vi "IMU Data Loop (RT RHIT's conflicted copy 2012-05-01).vi"() -> ()   [LabVIEW 2011]
uses:
  <vilib>/robotics/Controls/Compass Indicator/Compass Indicator.xctl
  <vilib>/Platform/TimedLoop/XDataNode/timing_clust.ctl
  <vilib>/Platform/TimedLoop/XDataNode/nitl_modes.ctl
  <vilib>/Platform/TimedLoop/XDataNode/wakeup.ctl
  <vilib>/Platform/TimedLoop/XDataNode/XDataNode.xnode
  <instrlib>/MicroStrain 3DM-GX1/MicroStrain 3DM-GX1.lvlib
  <vilib>/Platform/TimedLoop/XDataNode/XDNodeRunTimeDep.lvlib
panel:
  out "Waveform Chart 2":T1(graph)
  out "Waveform Chart":cluster{"Roll":dbl, "Pitch":dbl, "Yaw":dbl}(graph)
  in  "stop?":bool
  out "IMU Data":T2 {"Quaternion" format="%#.4g"; "Angular Rate"."Z-Axis Angular Rate" format="%#.4g"; "Angular Rate"."Y-Axis Angular Rate" format="%#.4g"; "Angular Rate"."X-Axis Angular Rate" format="%#.4g"; "Acceleration"."X-Axis Acceleration" format="%#.4g"; "Acceleration"."Y-Axis Acceleration" format="%#.4g"; "Acceleration"."Z-Axis Acceleration" format="%#.4g"; "Magnetic Field"."X-Axis Magnetic Field" format="%#.4g"; "Magnetic Field"."Y-Axis Magnetic Field" format="%#.4g"; "Magnetic Field"."Z-Axis Magnetic Field" format="%#.4g"; "Orientation Matrix" format="%#.4g"; "Position"."Yaw" format="%#.2f"; "Position"."Pitch" format="%#.1f"; "Position"."Roll" format="%#.1f"}
  in  "North Offset":dbl
  out "Compass Indicator":dbl(xcontrol)
  out "error out":errorcluster
  in  "Baud Rate":u32(ring)=115200 items=["19200"=19200, "38400"=38400, "115200"=115200]
  in  "Test Mode":bool
  in  "VISA resource name":refnum<visa-resource-name>="COM13"
  in  "Configure":bool
  out "Error Display":errorcluster
  in  "Enable Gyro-Stabilization (Enable)":bool=TRUE
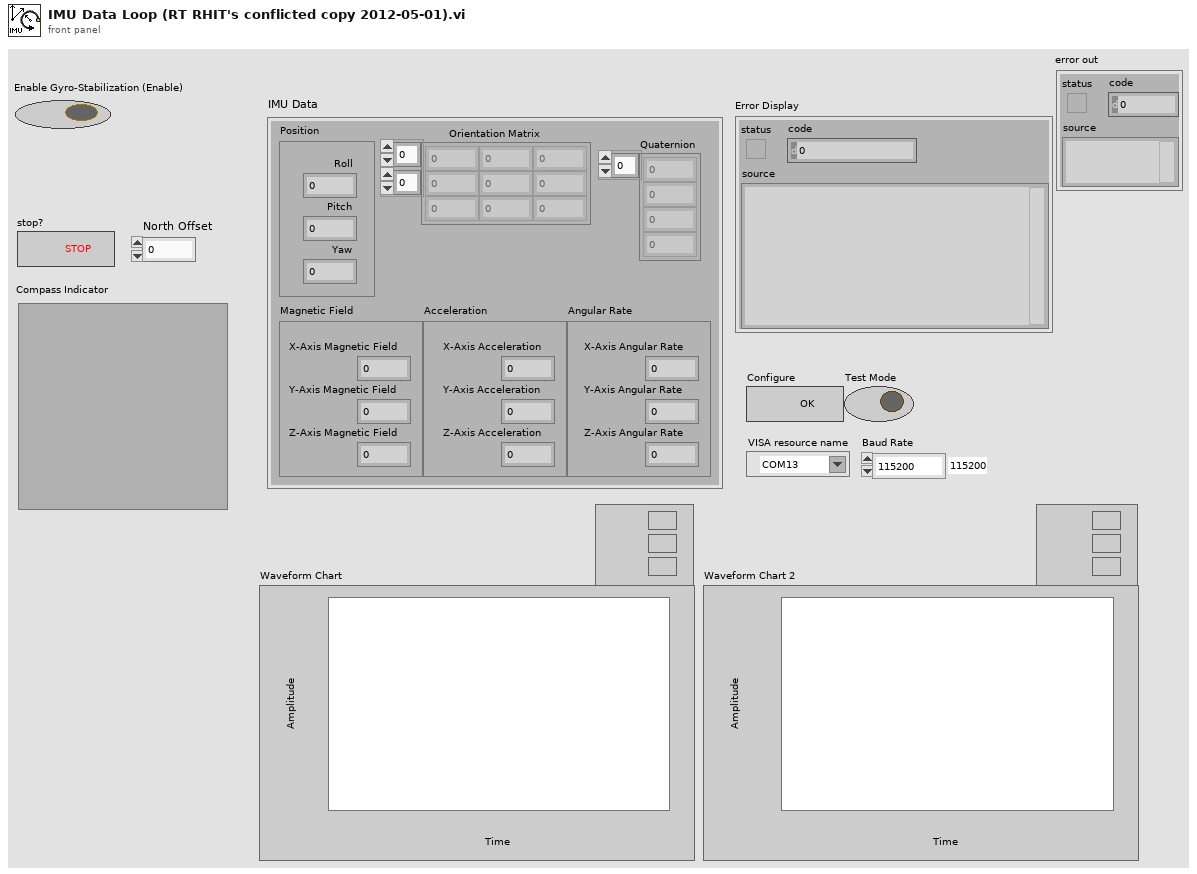
[diagram p1: front panel]
types:
  T1 = cluster{"X-Axis Magnetic Field":dbl, "Y-Axis Magnetic Field":dbl, "Z-Axis Magnetic Field":dbl}
  T2 = cluster{"Position":cluster{"Roll":dbl, "Pitch":dbl, "Yaw":dbl}, "Orientation Matrix":dbl[][], "Magnetic Field":cluster{"Z-Axis Magnetic Field":dbl, "Y-Axis Magnetic Field":dbl, "X-Axis Magnetic Field":dbl}, "Acceleration":cluster{"Z-Axis Acceleration":dbl, "Y-Axis Acceleration":dbl, "X-Axis Acceleration":dbl}, "Angular Rate":cluster{"X-Axis Angular Rate":dbl, "Y-Axis Angular Rate":dbl, "Z-Axis Angular Rate":dbl}, "Quaternion":dbl[]}
  T3 = typedef "XDNodeRunTimeDep.lvlib/timing_clust.ctl" = cluster{"Expected End [f-1]":u64, "Actual End [f-1]":u64, "Finished Late? [f-1]":bool, "Expected End [i-1]":u64, "Actual End [i-1]":u64, "Finished Late? [i-1]":bool, "Expected Start [i]":u64, "Actual Start [i]":u64, "Expected Start [f]":u64, "Actual Start [f]":u64, "Source Name":string, "Structure Name":string, "Period":i64, "Deadline":i64, "Offset":i64, "Start":i64, "Priority":i32, "Timeout":i32, "Mode":T4, "Wakeup Reason":T5, "Error":errorcluster, "Source Type":string, "Secondary Source Type":string, "Global End Time":u64, "Global Start Time":u64, "Frame Duration":u64, "Iteration Duration":u64, "Assigned CPU":i32, "I/O Scan Engine Mode":u32}
  T4 = typedef "XDNodeRunTimeDep.lvlib/nitl_modes.ctl" = enum32{"No Change", "Process missed periods, maintain original phase", "Discard missed periods, maintain original phase", "Process missed periods, ignore original phase", "Discard missed periods, ignore original phase"}
  T5 = typedef "XDNodeRunTimeDep.lvlib/wakeup.ctl" = enum32{"Normal", "Aborted", "Asynchronous wakeup", "Timing source error", "Timed loop error", "Timeout"}
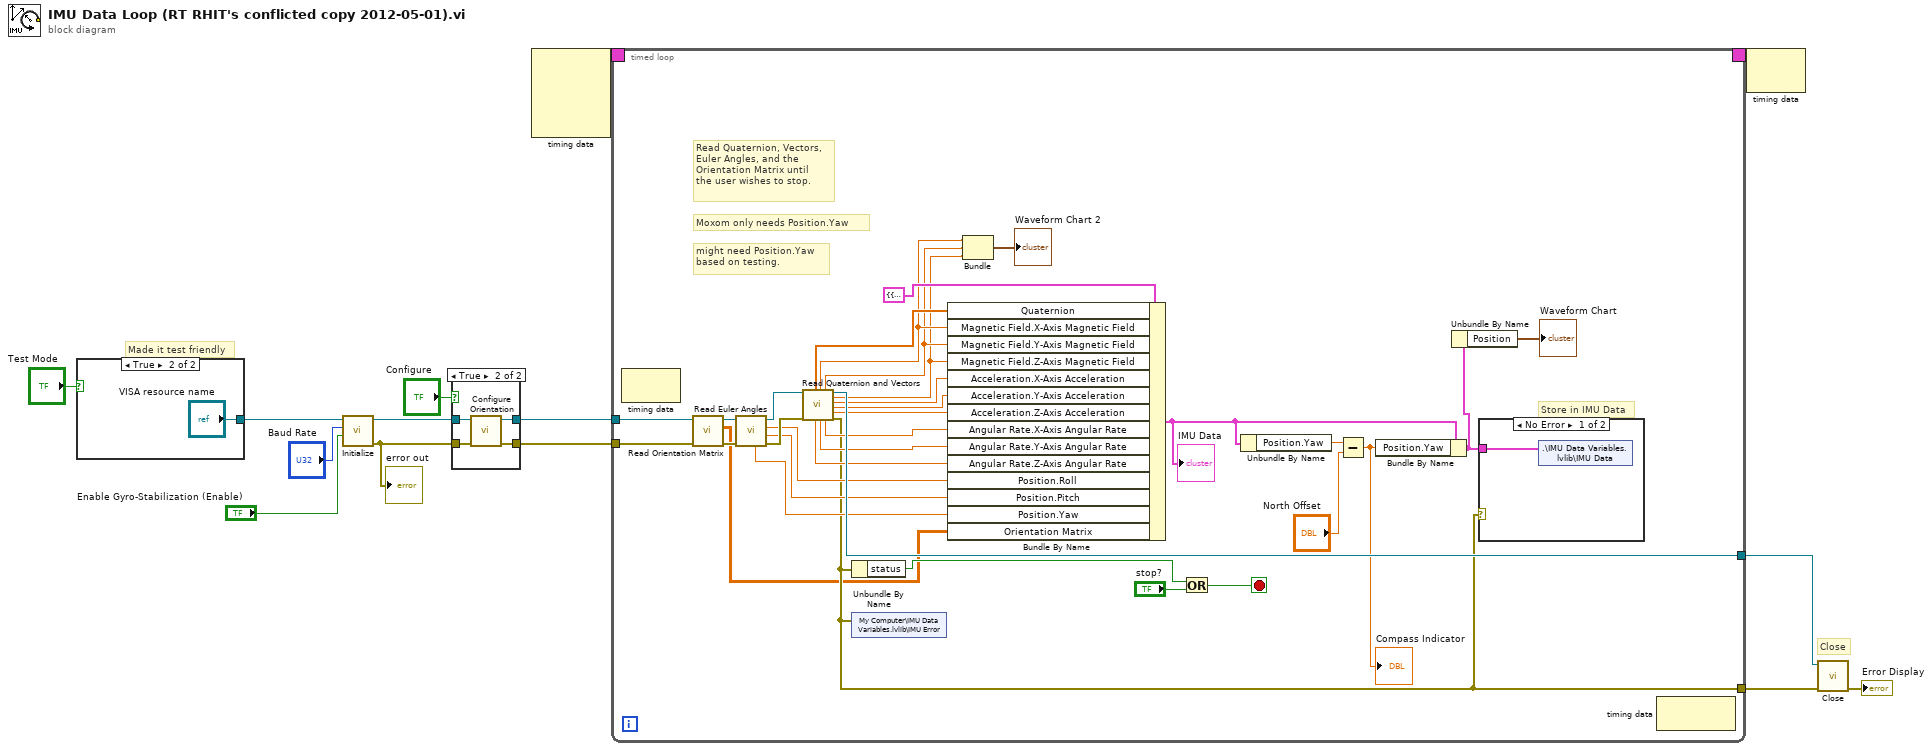
[diagram p0: block diagram]
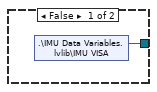
[diagram p3: hidden frame]
diagram:
  # "Made it test friendly"
  # "Close"
  n1 = case shown="True" "Test Mode" {
    tunnel: [w15 "VISA resource name"] -> w7
    frame False {
      n2 = shared-variable ".\\IMU Data Variables.lvlib\\IMU VISA"() -> (w15:refnum<visa-resource-name>)  [unwired: 1 in, 1 out]
    }
    frame True {
    }
  }
  n3 = call <instrlib>:"Initialize.vi"("Enable Gyro-Stabilization (True)"="Enable Gyro-Stabilization (Enable)", "Baud Rate (38400)"="Baud Rate", "VISA resource name"=w7) -> ("error out"=w11:errorcluster, "VISA resource name out"=w12:refnum<visa-resource-name>)  [unwired: 7 in]
  "error out" <- w11
  n4 = case shown="True" "Configure" {
    tunnel: w12 -> [w18 w22]
    tunnel: w11 -> [w17 w21]
    tunnel: [w18 w20] -> w2
    tunnel: [w17 w19] -> w1
    frame False {
    }
    frame True {
      n5 = call <instrlib>:"Configure Orientation.vi"("error in (no error)"=w21, "VISA resource name"=w22) -> ("error out"=w19:errorcluster, "VISA resource name out"=w20:refnum<visa-resource-name>)  [unwired: 8 in]
    }
  }
  n6 = node-c288() -> (w14:T3)  [unwired: 4 in]
  n7 = timed-loop {
    tunnel: [w36] -> w10
    tunnel: [w53] -> w9
    timing: w14 -> [_]
    timing-out: [_] -> w13
    tunnel: w2 -> [w30]
    tunnel: w1 -> [w29]
    stop <- w51 stop-if-true
    # "Moxom only needs Position.Yaw"
    # "Store in IMU Data"
    # "might need Position.Yaw\nbased on testing."
    # "Read Quaternion, Vectors,\nEuler Angles, and the\nOrientation Matrix until\nthe user wishes to stop."
    n8 = node-c288() -> ()  [unwired: 1 in, 1 out]
    n9 = call <instrlib>:"Read Orientation Matrix.vi"("error in (no error)"=w29, "VISA resource name"=w30) -> ("error out"=w54:errorcluster, "Orientation Matrix"=w35:dbl[][], "VISA resource name out"=w55:refnum<visa-resource-name>)  [unwired: 7 in]
    n10 = call <instrlib>:"Read Euler Angles.vi"("error in (no error)"=w54, "VISA resource name"=w55) -> ("error out"=w49:errorcluster, "Pitch"=w37:dbl, "Roll"=w39:dbl, "VISA resource name out"=w52:refnum<visa-resource-name>, "Yaw"=w38:dbl)  [unwired: 5 in]
    n11 = call <instrlib>:"Read Quaternion and Vectors.vi"("VISA resource name"=w52, "error in (no error)"=w49) -> ("Quaternion"=w46:dbl[], "Z-Axis Angular Rate"=w40:dbl, "X-Axis Magnetic Field"=w28:dbl, "Y-Axis Angular Rate"=w41:dbl, "Y-Axis Magnetic Field"=w27:dbl, "X-Axis Angular Rate"=w42:dbl, "VISA resource name out"=w53:refnum<visa-resource-name>, "Z-Axis Magnetic Field"=w26:dbl, "X-Axis Acceleration"=w45:dbl, "Y-Axis Acceleration"=w44:dbl, "Z-Axis Acceleration"=w43:dbl, "error out"=w36:errorcluster)  [unwired: 6 in]
    n12 = Unbundle By Name(w36) -> ("status"=w48:bool)
    n13 = shared-variable "My Computer\\IMU Data Variables.lvlib\\IMU Error"(w36) -> ()  [unwired: 1 in, 1 out]
    n14 = Bundle By Name(cluster=T2 {"Position"={"Roll"=0.0, "Pitch"=0.0, "Yaw"=0.0}, "Orientation Matrix"=[], "Magnetic Field"={"Z-Axis Magnetic Field"=0.0, "Y-Axis Magnetic Field"=0.0, "X-Axis Magnetic Field"=0.0}, "Acceleration"={"Z-Axis Acceleration"=0.0, "Y-Axis Acceleration"=0.0, "X-Axis Acceleration"=0.0}, "Angular Rate"={"X-Axis Angular Rate"=0.0, "Y-Axis Angular Rate"=0.0, "Z-Axis Angular Rate"=0.0}, "Quaternion"=[]} ("IMU Data"), "Quaternion"=w46, "Magnetic Field.X-Axis Magnetic Field"=w28, "Magnetic Field.Y-Axis Magnetic Field"=w27, "Magnetic Field.Z-Axis Magnetic Field"=w26, "Acceleration.X-Axis Acceleration"=w45, "Acceleration.Y-Axis Acceleration"=w44, "Acceleration.Z-Axis Acceleration"=w43, "Angular Rate.X-Axis Angular Rate"=w42, "Angular Rate.Y-Axis Angular Rate"=w41, "Angular Rate.Z-Axis Angular Rate"=w40, "Position.Roll"=w39, "Position.Pitch"=w37, "Position.Yaw"=w38, "Orientation Matrix"=w35) -> (w34:T2)
    "IMU Data" <- w34
    n15 = Bundle("X-Axis Magnetic Field"=w28, "Y-Axis Magnetic Field"=w27, "Z-Axis Magnetic Field"=w26) -> (→"Waveform Chart 2":T1)  [unwired: 1 in]
    n16 = Or(x=w48, y="stop?") -> (x .or. y?=w51:bool)
    n17 = Unbundle By Name(w34) -> ("Position.Yaw"=w33:dbl)
    n18 = Subtract(x=w33, y="North Offset") -> (x-y=w31:dbl)
    "Compass Indicator" <- w31
    n19 = Bundle By Name(cluster=w34, "Position.Yaw"=w31) -> (w24:T2)
    n20 = Unbundle By Name(w24) -> ("Position"=→"Waveform Chart":cluster{"Roll":dbl, "Pitch":dbl, "Yaw":dbl})
    n21 = case shown="No Error" w36 {
      tunnel: w24 -> [w58 _]
      frame No Error {
        n22 = shared-variable ".\\IMU Data Variables.lvlib\\IMU Data"(w58) -> ()  [unwired: 1 in, 1 out]
      }
      frame Error {
      }
    }
    n23 = node-c288() -> ()  [unwired: 1 in, 1 out]
  }
  n24 = node-c288(w13) -> ()  [unwired: 1 out]
  n25 = call <instrlib>:"Close.vi"("error in (no error)"=w10, "VISA resource name"=w9) -> ("error out"=→"Error Display":errorcluster)  [unwired: 9 in]
